vi "WS1021 MEMS Only ADI Read 24 DUT .vi"(6 "DUT Mask Mode (All)":T1=enum."All", 7 "FPGA":T2, 8 "Error In":errorcluster) -> (0 "Error Out":errorcluster, 3 "AD7747 Values":string[][](table))   [LabVIEW 2017]
uses:
  WS_VCAP Driver 1_49/Source/WSVCAP Shell/Type Defs/WSVCAP SHL FPGA Enum.ctl
  WS_VCAP Driver 1_49/Source/WSVCAP Shell/Type Defs/WSVCAP SHL I2C DUT Mask Mode Enum.ctl
  WS_VCAP Driver 1_49/Source/WSVCAP Shell/Type Defs/Cap and DAC Table Manager Operation Enum.ctl
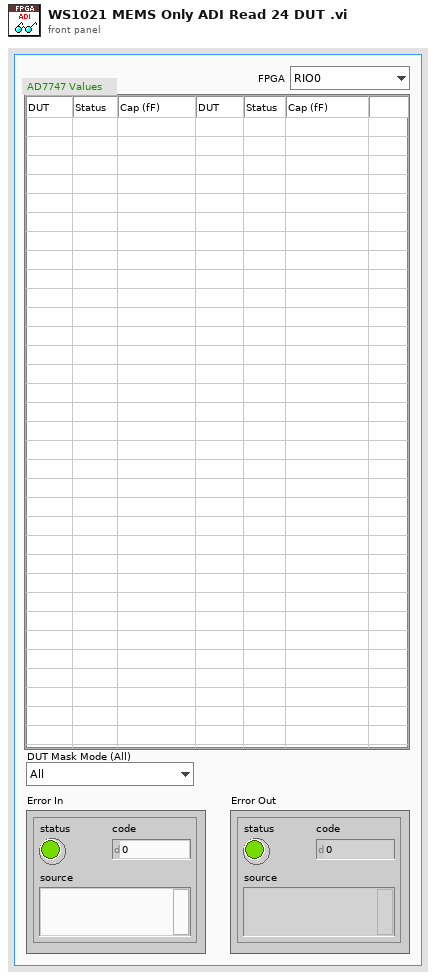
[diagram p1: front panel]
types:
  T1 = typedef "WSVCAP SHL I2C DUT Mask Mode Enum.ctl" = enum16{"Custom", "All"}
  T2 = typedef "WSVCAP SHL FPGA Enum.ctl" = enum16{"RIO0", "RIO1"}
  T3 = typedef "Cap and DAC Table Manager Operation Enum.ctl" = enum16{"Initialize", "Add Single DAC", "Add All DAC", "Add All DUT Single DAC", "Add All Cap", "Get Status"}
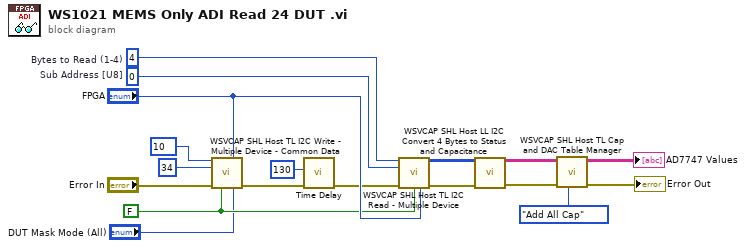
[diagram p0: block diagram]
diagram:
  w14 = u8 4  # Bytes to Read (1-4)
  w15 = u8 0  # Sub Address [U8]
  w8 = FALSE ("Log (T)")
  n1 = call "WSVCAP SHL Host TL I2C Write - Multiple Device - Common Data.vi"("Sub Address"=u8 10, "FPGA"="FPGA", "Data Out [U8]"=u8 34, "error in"="Error In", "Log (T)"=w8, "DUT Mask Mode (All)"="DUT Mask Mode (All)") -> ("error out"=w11:errorcluster)  [unwired: 9 in]
  n2 = call "Time Delay.vi"("Error In"=w11, "Delay(ms)"=u32 130) -> ("Error Out"=w9:errorcluster)  [unwired: 9 in]
  n3 = call "WSVCAP SHL Host TL I2C Read - Multiple Device.vi"("Bytes to Read (1-4)"=w14, "Sub Address [U8]"=w15, "error in"=w9, "Log (T)"=w8, "FPGA"="FPGA") -> ("C:1-24 Read Data [U8]"=w13:u8[][], "error out"=w4:errorcluster)  [unwired: 9 in]
  n4 = call "WSVCAP SHL Host LL I2C Convert 4 Bytes to Status and Capacitance.vi"("C:1-24 Read Data [U8]"=w13) -> ("AD7747 Values"=w5:string[][])  [unwired: 14 in]
  n5 = call "WSVCAP SHL Host TL Cap and DAC Table Manager.vi"("Operation"=Cap_and_DAC_Table_Manager_Operation_Enum."Add All Cap", "Error In"=w4, "Data In"=w5) -> ("Error Out"=→"Error Out":errorcluster, "Table Out"=→"AD7747 Values":string[][])  [unwired: 7 in]
